vi "PictureCrop.vi"() -> ()   [LabVIEW 2017]
uses:
  <vilib>/Utility/config.llb/Read Key (String).vi
  <vilib>/vision/NI_Vision_Development_Module.lvlib
  <vilib>/vision/driver/NI_Vision_Acquisition_Software.lvlib
  <vilib>/Utility/config.llb/NI_LVConfig.lvlib
panel:
  in  "cancel":bool
  in  "Done":bool
  in  "Snapshot":bool
  out "Image":T1(plugin-control)
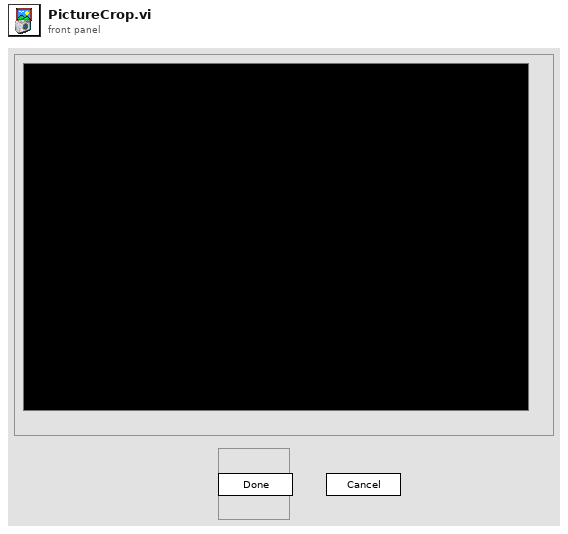
[diagram p1: front panel]
types:
  T1 = typedef "IMAQ Image.ctl" = refnum<image>
  T2 = typedef "Image Type" = u32
  T3 = typedef "NI_LVConfig.lvlib/Config Data RefNum.ctl" = refnum<k1>
  T4 = typedef "IMAQdx.ctl" = refnum<k21>
  T5 = cluster{"Global Rectangle":i32[], "Contours":cluster{"Contour Type":u32, "ROI Type":u32, "Points":i32[]}[]}
  T6 = typedef "IMAQ Rectangle" = cluster{"Left":i32, "Top":i32, "Right":i32, "Bottom":i32, "Rotation":dbl}
  T7 = cluster{"Left":i32, "Top":i32, "Right":i32, "Bottom":i32, "Rotation":i32}
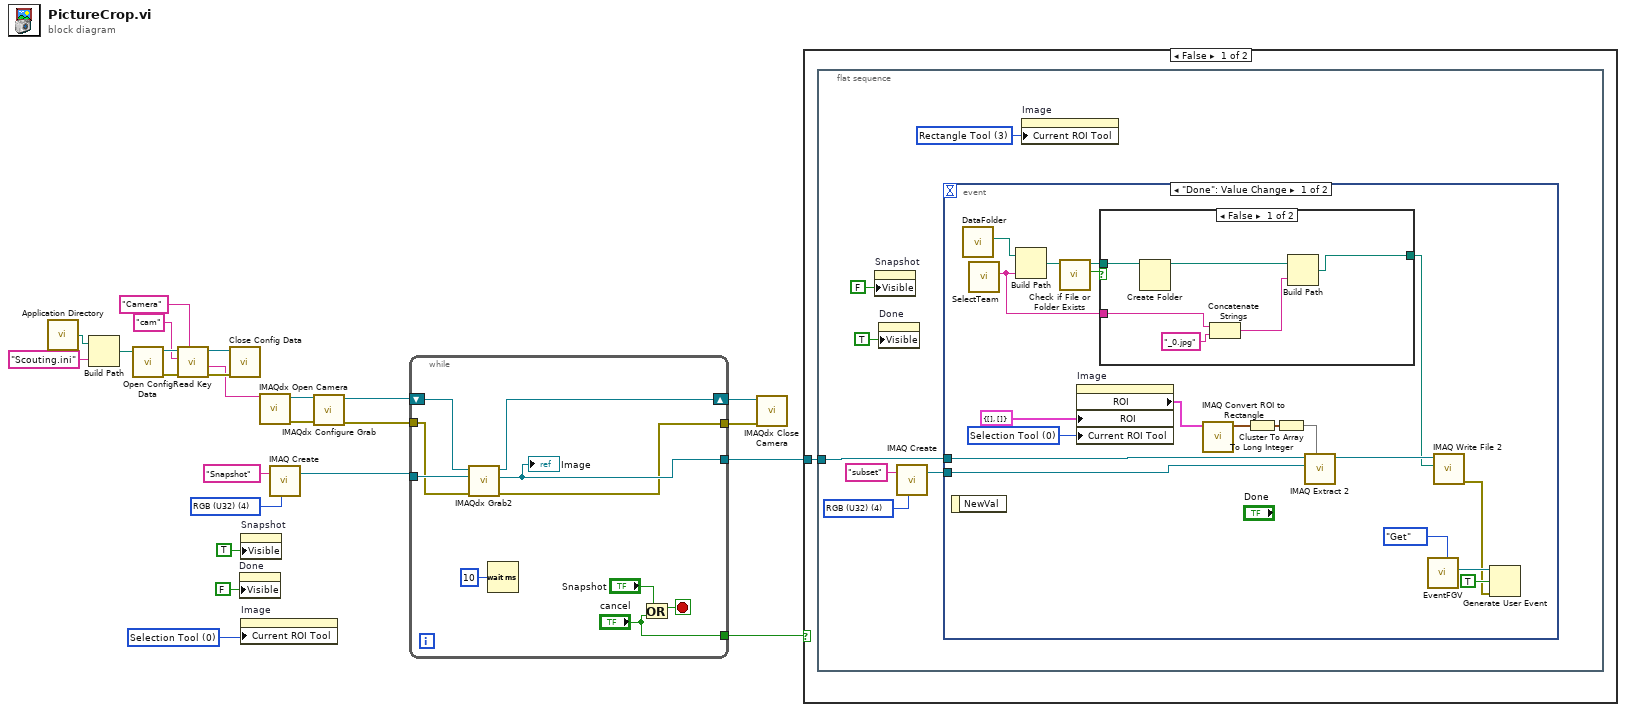
[diagram p0: block diagram]
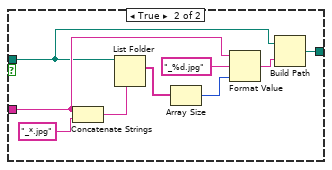
[diagram p2: hidden frame]
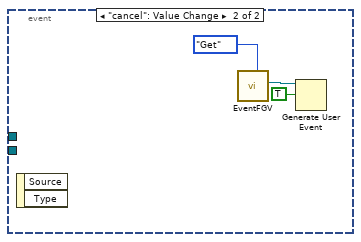
[diagram p3: hidden frame]
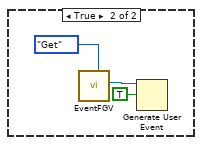
[diagram p4: hidden frame]
diagram:
  w16 = u32 0 items=["Zoom Tool"=8, "Selection Tool"=0, "Pan Tool"=9, "Point Tool"=1, "Line Tool"=2, "Rectangle Tool"=3, "Rotated Rectangle Tool"=12, "Polyline Tool"=10, "Polygon Tool"=5, "Freehand Tool"=11, "Closed Freehand Tool"=6, "Ellipse Tool"=4, "Annulus Tool"=7] ("Current ROI Tool")
  w24 = T2 4 items=["Grayscale (U8)", "Grayscale (I16)", "Grayscale (SGL)", "Complex (CSG)", "RGB (U32)", "HSL (U32)", "RGB (U64)", "Grayscale (U16)"] ("Image Type")
  n1 = call <vilib>:"Application Directory.vi"() -> ("Application Directory"=w12:path)
  n2 = Build Path(base path=w12, name or relative path="Scouting.ini") -> (appended path=w10:path)
  n3 = call <vilib>:"Open Config Data.vi"("configuration file path"=w10) -> ("error out"=w9:errorcluster, "refnum"=w8:T3)  [unwired: 8 in, 1 out]
  n4 = call-poly <vilib>:"Read Key.vi"("section"="Camera", "error in (no error)"=w9, "key"="cam", "refnum"=w8) -> ("error out"=w5:errorcluster, "value"=w3:string, "refnum out"=w4:T3)  [unwired: 4 in, 1 out]
  n5 = call <vilib>:"Close Config Data.vi"("error in (no error)"=w5, "refnum"=w4) -> ()  [unwired: 8 in, 2 out]
  n6 = property on="Done" class="Bool"("Visible"=FALSE) -> ()  [unwired: 2 in, 2 out]
  n7 = property on="Snapshot" class="Bool"("Visible"=TRUE) -> ()  [unwired: 2 in, 2 out]
  n8 = property on="Image" class="ImageControl"("Current ROI Tool"=w16) -> ()  [unwired: 2 in, 2 out]
  n9 = call <vilib>:"IMAQdx Open Camera.vi"("Session In"=w3) -> ("error out"=w15:errorcluster, "Session Out"=w22:T4)  [unwired: 9 in]
  n10 = call "IMAQ Create"("Image Name"="Snapshot", "Image Type"=w24) -> ("New Image"=w21:T1)  [unwired: 3 in, 1 out]
  n11 = call <vilib>:"IMAQdx Configure Grab.vi"("error in"=w15, "Session In"=w22) -> ("error out"=w14:errorcluster, "Session Out"=w23:T4)  [unwired: 8 in]
  n12 = while {
    shift-right: [w32] -> w19
    shift-left: w23 -> [w33]
    tunnel: w21 -> [w34]
    tunnel: [w29] -> w18
    tunnel: w14 -> [w28]
    tunnel: [w27] -> w13
    tunnel: ["cancel"] -> w2
    stop <- w26 stop-if-true
    n13 = call <vilib>:"IMAQdx Grab2.vi"("error in"=w28, "Image In"=w34, "Session In"=w33) -> ("error out"=w27:errorcluster, "Image Out"=w29:T1, "Session Out"=w32:T4)  [unwired: 5 in, 1 out]
    "Image" <- w29
    n14 = Wait (ms)(milliseconds to wait=u32 10) -> ()  [unwired: 1 out]
    n15 = Or(x="Snapshot", y="cancel") -> (x .or. y?=w26:bool)
  }
  n16 = call <vilib>:"IMAQdx Close Camera.vi"("error in"=w13, "Session In"=w19) -> ()  [unwired: 9 in, 1 out]
  n17 = case shown="False" w2 {
    tunnel: w18 -> [w35 _]
    frame False {
      n18 = flat-sequence {
        tunnel: w35 -> [w38]
        frame #0 {
          w39 = u32 3 items=["Zoom Tool"=8, "Selection Tool"=0, "Pan Tool"=9, "Point Tool"=1, "Line Tool"=2, "Rectangle Tool"=3, "Rotated Rectangle Tool"=12, "Polyline Tool"=10, "Polygon Tool"=5, "Freehand Tool"=11, "Closed Freehand Tool"=6, "Ellipse Tool"=4, "Annulus Tool"=7] ("Current ROI Tool")
          w41 = T2 4 items=["Grayscale (U8)", "Grayscale (I16)", "Grayscale (SGL)", "Complex (CSG)", "RGB (U32)", "HSL (U32)", "RGB (U64)", "Grayscale (U16)"] ("Image Type")
          n19 = property on="Snapshot" class="Bool"("Visible"=FALSE) -> ()  [unwired: 2 in, 2 out]
          n20 = property on="Done" class="Bool"("Visible"=TRUE) -> ()  [unwired: 2 in, 2 out]
          n21 = call "IMAQ Create"("Image Name"="subset", "Image Type"=w41) -> ("New Image"=w40:T1)  [unwired: 3 in, 1 out]
          n22 = event shown="[0] \"Done\": Value Change" {
            selector: _ -> [_ _]
            dyn-events: _ -> [_ _]
            timeout: _ -> [_ _]
            tunnel: w38 -> [w54 _]
            tunnel: w40 -> [w57 _]
            event "Done": Value Change {
              w55 = u32 0 items=["Zoom Tool"=8, "Selection Tool"=0, "Pan Tool"=9, "Point Tool"=1, "Line Tool"=2, "Rectangle Tool"=3, "Rotated Rectangle Tool"=12, "Polyline Tool"=10, "Polygon Tool"=5, "Freehand Tool"=11, "Closed Freehand Tool"=6, "Ellipse Tool"=4, "Annulus Tool"=7] ("Current ROI Tool")
              n23 = event-data() -> ()  [unwired: 1 in, 1 out]
              n24 = call "DataFolder.vi"() -> ("appended path"=w48:path)  [unwired: 11 in]
              n25 = call "SelectTeam.vi"() -> ("Selected Team"=w44:string)  [unwired: 11 in]
              n26 = Build Path(base path=w48, name or relative path=w44) -> (appended path=w47:path)
              n27 = call <vilib>:"Check if File or Folder Exists.vi"("path"=w47) -> ("file or folder exists?"=w45:bool, "dup path"=w46:path)  [unwired: 8 in, 1 out]
              n28 = property on="Image" class="ImageControl"("ROI"=T5 {"Global Rectangle"=[], "Contours"=[]}, "Current ROI Tool"=w55) -> ("ROI"=w61:T5)  [unwired: 2 in, 2 out]
              n29 = case shown="False" w45 {
                tunnel: w46 -> [w67 w69]
                tunnel: w44 -> [w65 w72]
                tunnel: [w62 w68] -> w43
                frame False {
                  n30 = Create Folder(path (use dialog)=w67) -> (created path=w64:path)  [unwired: 2 in, 2 out]
                  n31 = Concatenate Strings(w65, "_0.jpg" ("format string")) -> (w63:string)
                  n32 = Build Path(base path=w64, name or relative path=w63) -> (appended path=w62:path)
                }
                frame True {
                  n33 = Concatenate Strings(w72, "_*.jpg" ("string")) -> (w75:string)
                  n34 = List Folder(path=w69, pattern=w75) -> (filenames=w74:string[])  [unwired: 2 in, 3 out]
                  n35 = Array Size(array=w74) -> (size(s)=w73:i32)
                  n36 = Format Value(string ("")=w72, format string="_%d.jpg", value (0)=w73) -> (output string=w70:string)
                  n37 = Build Path(base path=w69, name or relative path=w70) -> (appended path=w68:path)
                }
              }
              n38 = call "IMAQ Convert ROI to Rectangle"("ROI Descriptor"=w61) -> ("Rectangle"=w60:T6)  [unwired: 8 in, 1 out]
              n39 = To Long Integer(number=w60) -> (32bit integer=w59:T7)
              n40 = Cluster To Array(cluster=w59) -> (array=w58:i32[])
              n41 = call "IMAQ Extract 2"("Optional Rectangle"=w58, "Image Dst"=w57, "Image Src"=w54) -> ("Image Dst Out"=w49:T1)  [unwired: 7 in, 1 out]
              n42 = call "EventFGV.vi"("Action"=enum16{"Set", "Get"}."Get") -> ("user event out"=w53:refnum<user-event>)  [unwired: 10 in]
              n43 = call-poly "IMAQ Write File 2"("File Path"=w43, "Image"=w49) -> ("error out"=w50:errorcluster)  [unwired: 8 in, 1 out]
              n44 = Generate User Event(user event=w53, event data cluster=TRUE ("event data"), error in=w50) -> ()  [unwired: 1 in, 2 out]
            }
            event "cancel": Value Change {
              n45 = event-data() -> ()  [unwired: 1 in, 2 out]
              n46 = call "EventFGV.vi"("Action"=enum16{"Set", "Get"}."Get") -> ("user event out"=w79:refnum<user-event>)  [unwired: 10 in]
              n47 = Generate User Event(user event=w79, event data cluster=TRUE ("event data")) -> ()  [unwired: 2 in, 2 out]
            }
          }
          n48 = property on="Image" class="ImageControl"("Current ROI Tool"=w39) -> ()  [unwired: 2 in, 2 out]
        }
      }
    }
    frame True {
      n49 = call "EventFGV.vi"("Action"=enum16{"Set", "Get"}."Get") -> ("user event out"=w82:refnum<user-event>)  [unwired: 10 in]
      n50 = Generate User Event(user event=w82, event data cluster=TRUE ("event data")) -> ()  [unwired: 2 in, 2 out]
    }
  }
